vi "Test Finding Tests at Empty Path Throws Error.vi"(8 "error in (no error)":errorcluster, 11 "Test Finder Test in":refnum<class "Test Finder Test.lvclass">) -> (0 "error out":errorcluster, 3 "Test Finder Test out":refnum<class "Test Finder Test.lvclass">)   [LabVIEW 2020, in "LUnit Tests.lvlib" / "Test Finder Test.lvclass"]
uses:
  Test Finder Test.lvclass
  C:/Program Files (x86)/National Instruments/LabVIEW 2020/vi.lib/Astemes/LUnit/Test Case.lvclass
  Test Finder Test.lvclass/Test Finder Test.ctl
  <vilib>/Astemes/LUnit/Test Case.lvclass/Test Case.ctl
  <vilib>/Astemes/LUnit/LUnit Assertion Result.lvclass/LUnit Assertion Result.ctl
  <vilib>/Astemes/LUnit/LUnit Test Case Result.lvclass/LUnit Test Case Result.ctl
  <vilib>/Astemes/LUnit/LUnit Method Result.lvclass/LUnit Method Result.ctl
  <vilib>/Astemes/LUnit/Palette/Fail.vi
  <vilib>/Astemes/LUnit/Palette/Pass.vi
  <vilib>/Astemes/LUnit/Set Assertion Type.vi
  <vilib>/Astemes/LUnit/Add test result.vi
  <vilib>/Astemes/LUnit/LUnit Write Passed.vi
  <vilib>/Astemes/LUnit/LUnit Write Message.vi
  <vilib>/Astemes/LUnit/LUnit Write Description.vi
  <vilib>/Astemes/LUnit/LUnit Write Assertion Type.vi
  <vilib>/Astemes/LUnit/LUnit Record Assertion Result.vi
  <vilib>/Astemes/LUnit/LUnit Aggregate Assertion Results.vi
  <vilib>/Astemes/LUnit/Assertion Result/LUnit Read Status.vi
  <vilib>/Astemes/LUnit/LUnit Read Message.vi
  <vilib>/Astemes/LUnit/LUnit Read Description.vi
  <vilib>/Astemes/LUnit/Method Result/LUnit Merge Status.vi
  <vilib>/Astemes/LUnit/LUnit Concatenate result strings.vi
  source/Framework/Helper Classes/Test Finder/Test Finder.lvclass
  <vilib>/Astemes/LUnit/LUnit Assertion Result.lvclass
  <vilib>/Astemes/LUnit/Test Case.lvclass
  C:/Git/astemes-lunit/tests/Test Finder/Test Finder Test.lvclass
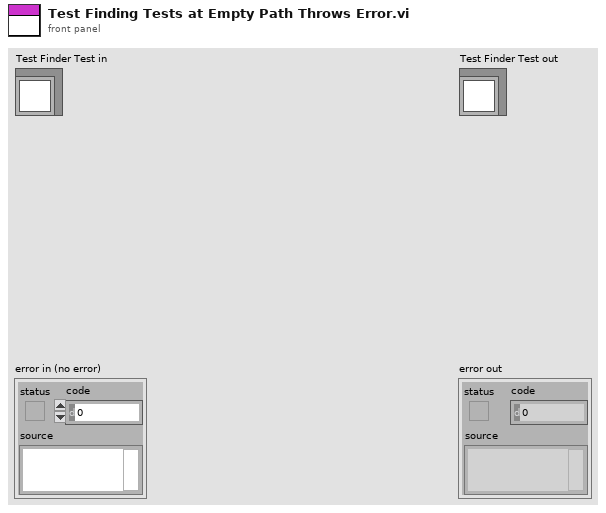
[diagram p1: front panel]
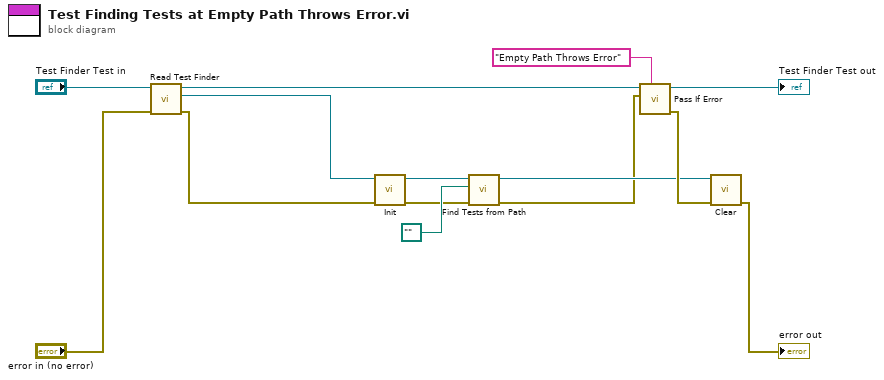
[diagram p0: block diagram]
diagram:
  n1 = call "Read Test Finder.vi"("error in (no error)"="error in (no error)", "Test Finder In"="Test Finder Test in") -> ("error out"=w5:errorcluster, "Test Finder.lvclass"=w6:refnum<class "Test Finder.lvclass">, "Test Finder Out"=w12:refnum<class "Test Finder Test.lvclass">)  [unwired: 7 in]
  n2 = call-dynamic "Init.vi"("error in (no error)"=w5, "Test Finder in"=w6) -> ("error out"=w7:errorcluster, "Test Finder out"=w8:refnum<class "Test Finder.lvclass">)  [unwired: 8 in]
  n3 = call-dynamic "Find Tests from Path.vi"("error in (no error)"=w7, "Project or Class Path"=path "", "Test Case Finder In"=w8) -> ("error out"=w2:errorcluster, "Test Case Finder Out"=w3:refnum<class "Test Finder.lvclass">)  [unwired: 7 in]
  n4 = call <vilib>:"Pass If Error.vi"("Description"="Empty Path Throws Error", "Assert error"=w2, "LUnit Test Case In"=w12) -> ("error out"=w4:errorcluster, "LUnit Test Case Out"=→"Test Finder Test out":refnum<class "Test Finder Test.lvclass">)  [unwired: 7 in]
  n5 = call "Clear.vi"("error in (no error)"=w4, "Test Finder in"=w3) -> ("error out"=→"error out":errorcluster)  [unwired: 8 in, 1 out]
